vi "Servo_enable.vi"(8 "error in":errorcluster, 9 "Enable 2":bool=TRUE, 10 "Enable":bool=TRUE) -> (0 "error out":errorcluster)   [LabVIEW 2009, in "Servo.lvlib"]
uses:
  Servo.lvlib
  PWM/PWM_Name.ctl
  PWM.lvlib
  FPGA.lvlib
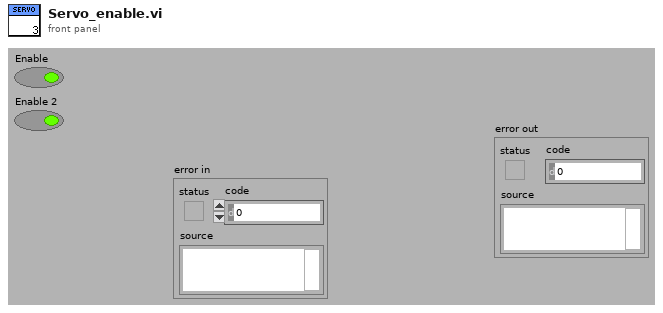
[diagram p1: front panel]
types:
  T1 = typedef "PWM.lvlib/PWM_Name.ctl" = u16
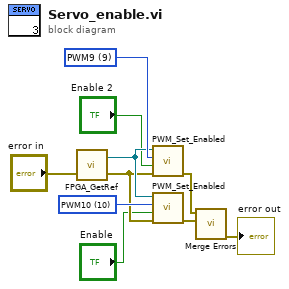
[diagram p0: block diagram]
diagram:
  w6 = T1 10 items=["Invalid"=0, "PWM1"=1, "PWM2"=2, "PWM9"=9, "PWM10"=10] ("PWM_in")
  w7 = T1 9 items=["Invalid"=0, "PWM1"=1, "PWM2"=2, "PWM9"=9, "PWM10"=10] ("PWM_in")
  n1 = call "FPGA_GetRef.vi"("error in (no error)"="error in") -> ("error out"=w3:errorcluster, "FPGA_Ref"=w5:refnum<k20>)  [unwired: 1 in]
  n2 = call "PWM_Set_Enabled.vi"("error in"=w3, "Enable"="Enable 2", "PWM_in"=w7, "FPGA_Ref_in"=w5) -> ("error out"=w9:errorcluster)  [unwired: 5 in, 2 out]
  n3 = call "PWM_Set_Enabled.vi"("error in"=w3, "Enable"="Enable", "PWM_in"=w6, "FPGA_Ref_in"=w5) -> ("error out"=w8:errorcluster)  [unwired: 5 in, 2 out]
  n4 = call <vilib>:"Merge Errors.vi"("error in 2 (no error)"=w8, "error in 1 (no error)"=w9) -> ("error out"=→"error out":errorcluster)  [unwired: 5 in]
